vi "PutRow Example.vi"() -> ()   [LabVIEW 2010]
uses:
  <vilib>/builds/MDSplus/MDSplus/MDSplus.lvlib
panel:
  in  "Event Name":string="my_tree"
  in  "Node Path":string=":SIG_0"
  in  "Shot":i32=-1
  in  "Tree Name":string="my_tree"
  out "Waveform Chart":dbl(graph)
  in  "stop":bool
  in  "phase":dbl
  in  "amplitude":dbl=5.0
  in  "frequency":dbl=1.1
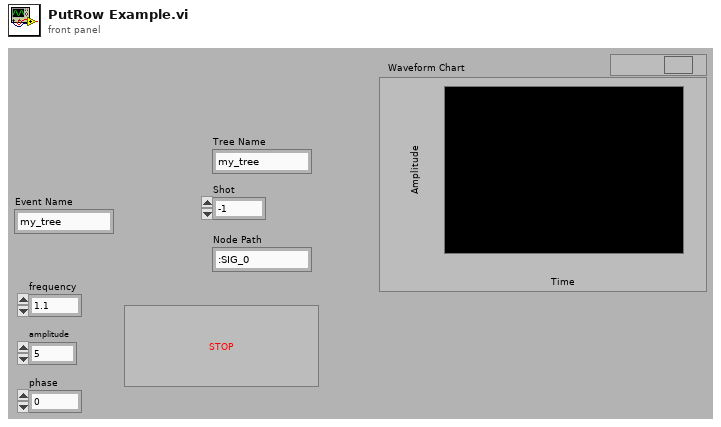
[diagram p1: front panel]
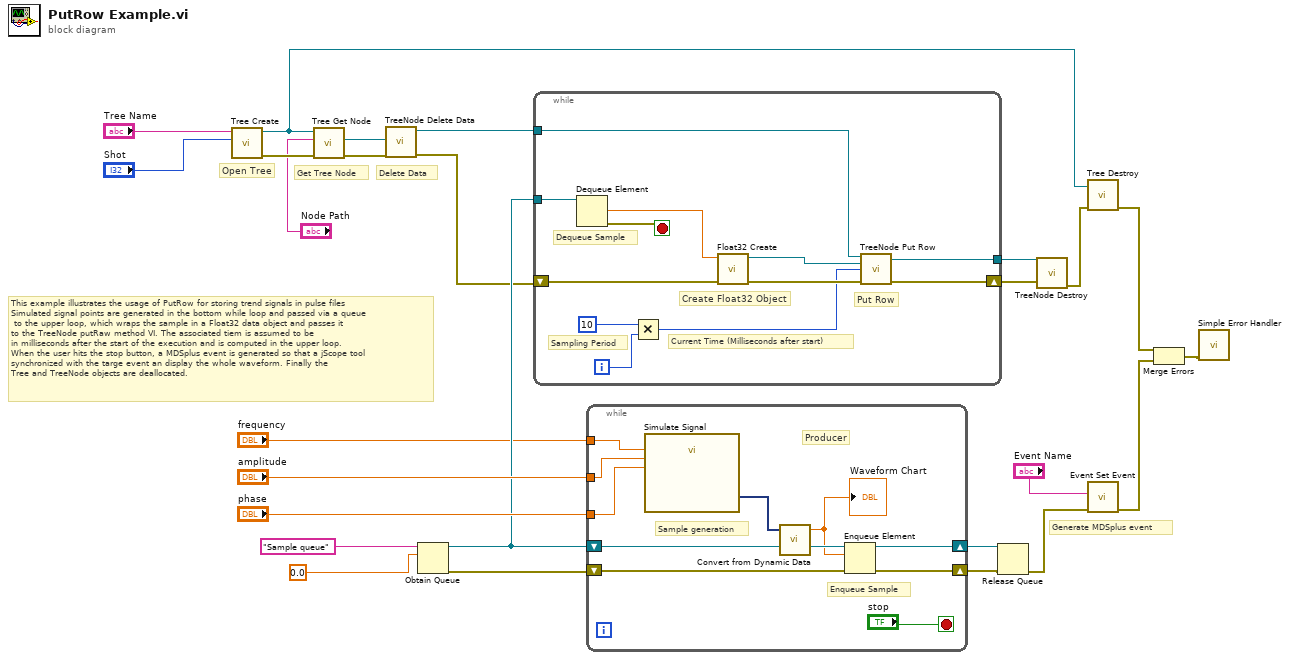
[diagram p0: block diagram]
diagram:
  # "This example illustrates the usage of PutRow for storing trend signals in pulse files\nSimulated signal points are generated in the bottom while loop and passed via a queue\n to the upper loop, which wraps the sample in a Float32 data object and passes it\nto the TreeNode putRaw method VI. The associated tiem is assumed to be\nin milliseconds after the start of the execution and is computed in the upper loop.\nWhen the user hits the stop button, a MDSplus event is generated so that a jScope tool\nsynchronized with the targe event an display the whole waveform. Finally the\nTree and TreeNode objects are deallocated."
  # "Generate MDSplus event"
  # "Delete Data"
  # "Get Tree Node"
  # "Open Tree"
  n1 = call <vilib>:"Tree Create.vi"("Shot"="Shot", "Name"="Tree Name") -> ("error out"=w20:errorcluster, "Tree DVR out"=w5:refnum<data-value>)  [unwired: 8 in]
  n2 = call <vilib>:"Tree Get Node.vi"("error in (no error)"=w20, "Path"="Node Path", "Tree DVR in"=w5) -> ("error out"=w17:errorcluster, "Node out"=w12:refnum<data-value>)  [unwired: 6 in, 1 out]
  n3 = call <vilib>:"TreeNode Delete Data.vi"("error in (no error)"=w17, "TreeNode DVR in"=w12) -> ("error out"=w14:errorcluster, "TreeNode DVR out"=w4:refnum<data-value>)  [unwired: 8 in]
  n4 = Obtain Queue(name (unnamed)="Sample queue", element data type=0.0 ("Numeric")) -> (queue out=w22:refnum<queue>, error out=w21:errorcluster)  [unwired: 3 in, 1 out]
  n5 = while {
    tunnel: w22 -> [w38]
    shift-right: [w34] -> w10
    shift-left: w14 -> [w33]
    tunnel: [w31] -> w9
    tunnel: w4 -> [w28]
    i -> [w37]
    stop <- w30 stop-if-true
    # "Sampling Period"
    # "Put Row"
    # "Current Time (Milliseconds after start)"
    # "Create Float32 Object"
    # "Dequeue Sample"
    n6 = Dequeue Element(queue=w38) -> (element=w36:dbl, error out=w30:errorcluster)  [unwired: 2 in, 2 out]
    n7 = Multiply(x=10, y=w37) -> (x*y=w32:i32)
    n8 = call <vilib>:"Float32 Create.vi"("error in (no error)"=w33, "SGL in"=w36) -> ("error out"=w35:errorcluster, "Float32 DVR out"=w29:refnum<data-value>)  [unwired: 8 in]
    n9 = call <vilib>:"TreeNode Put Row.vi"("TreeNode DVR in"=w28, "Row Data"=w29, "Time"=w32, "error in (no error)"=w35) -> ("TreeNode DVR out"=w31:refnum<data-value>, "error out"=w34:errorcluster)  [unwired: 10 in]
  }
  n10 = while {
    tunnel: "frequency" -> [w44]
    tunnel: "amplitude" -> [w43]
    tunnel: "phase" -> [w42]
    shift-right: [w46] -> w3
    shift-left: w22 -> [w48]
    shift-right: [w45] -> w2
    shift-left: w21 -> [w47]
    stop <- "stop" stop-if-true
    # "Sample generation"
    # "Enqueue Sample"
    # "Producer"
    n11 = call "Simulate Signal"("Frequency"=w44, "Amplitude"=w43, "Phase"=w42) -> ("Sine"=w41:dynamicdata)  [unwired: 11 in, 1 out]
    n12 = call "Convert from Dynamic Data"("Dynamic Data Type"=w41) -> ("Scalar"=w39:dbl)  [unwired: 3 in]
    "Waveform Chart" <- w39
    n13 = Enqueue Element(queue=w48, element=w39, error in (no error)=w47) -> (queue out=w46:refnum<queue>, error out=w45:errorcluster)  [unwired: 1 in, 1 out]
  }
  n14 = Release Queue(queue=w3, error in (no error)=w2) -> (error out=w1:errorcluster)  [unwired: 1 in, 2 out]
  n15 = call <vilib>:"TreeNode Destroy.vi"("error in (no error)"=w10, "TreeNode DVR in"=w9) -> ("error out"=w8:errorcluster)  [unwired: 9 in]
  n16 = call <vilib>:"Tree Destroy.vi"("error in (no error)"=w8, "Tree DVR in"=w5) -> ("error out"=w7:errorcluster)  [unwired: 9 in]
  n17 = call <vilib>:"Event Set Event.vi"("error in (no error)"=w1, "Event name"="Event Name") -> ("error out"=w6:errorcluster)  [unwired: 8 in, 1 out]
  n18 = Merge Errors(w7, w6) -> (w13:errorcluster)
  n19 = call <vilib>:"Simple Error Handler.vi"("error in (no error)"=w13) -> ()  [unwired: 4 in, 5 out]
